vi "P32_Servo.vi"() -> ()   [LabVIEW 2022 SP3]
panel:
  in  "stop":bool
  # "P32_Servo"
  # "Equipo C\nJairo Issac García López\nRodolfo Durón Hernandez\nRoberto Carlos Herrera Pérez\nSebastián Rodríguez Posada"
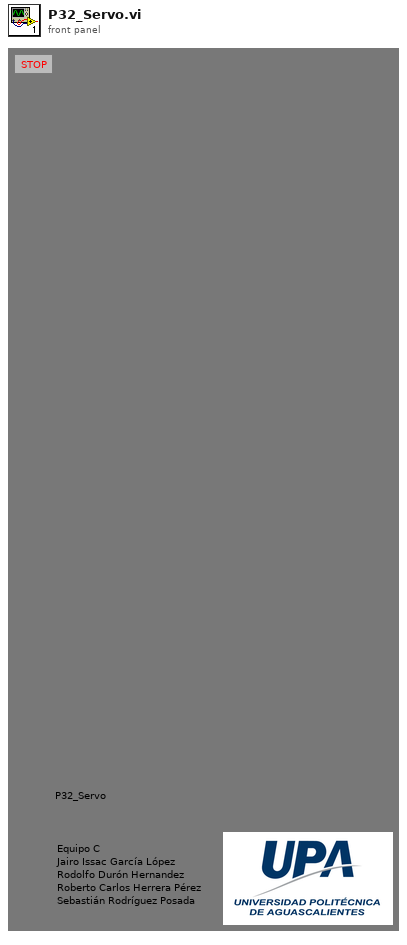
[diagram p1: front panel]
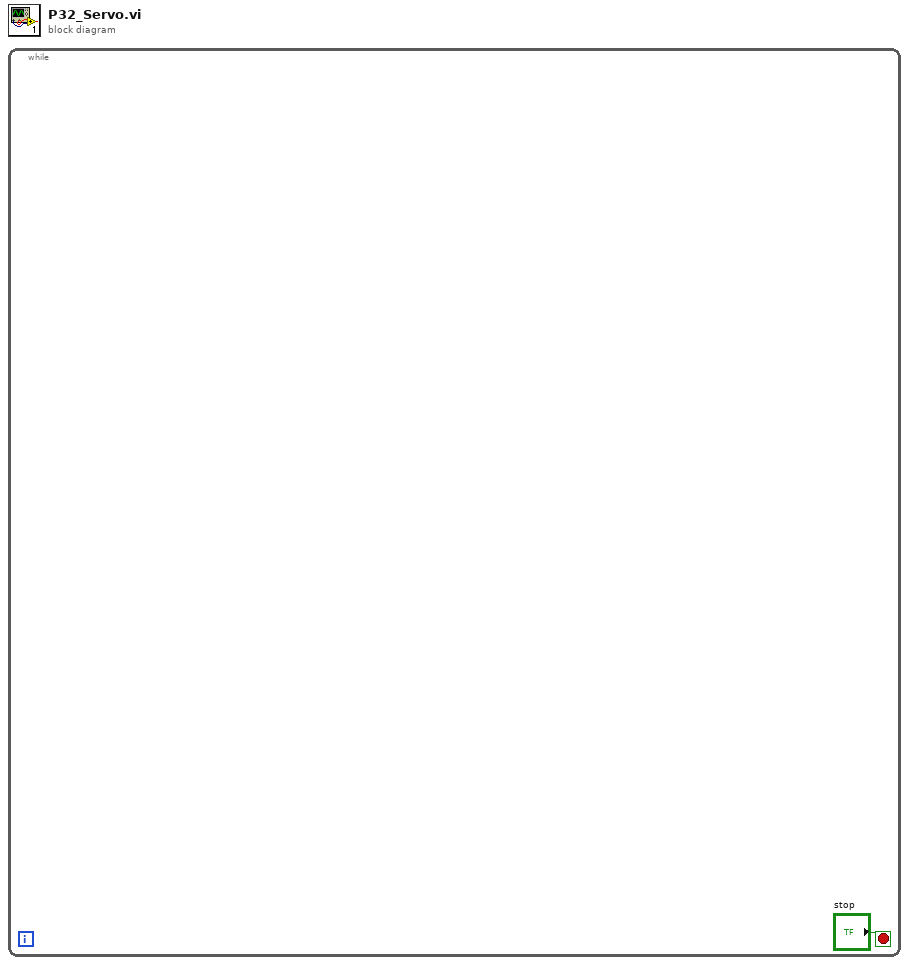
[diagram p0: block diagram]
diagram:
  n1 = while {
    stop <- "stop" stop-if-true
  }
